vi "FlipAngleFunction.vi"(11 "AngleInput":dbl) -> (3 "AngleFlipped":dbl)   [LabVIEW 2018]
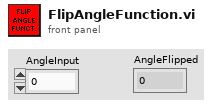
[diagram p1: front panel]
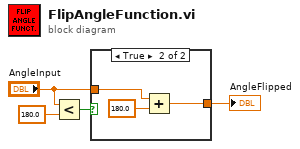
[diagram p0: block diagram]
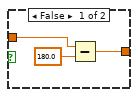
[diagram p2: hidden frame]
diagram:
  n1 = Less?(x="AngleInput", y=180.0) -> (x < y?=w3:bool)
  n2 = case shown="True" w3 {
    tunnel: "AngleInput" -> [w5 w10]
    tunnel: [w6 w8] -> w1
    frame False {
      n3 = Subtract(x=w5, y=180.0) -> (x-y=w6:dbl)
    }
    frame True {
      n4 = Add(x=w10, y=180.0) -> (x+y=w8:dbl)
    }
  }
  "AngleFlipped" <- w1
